vi "Assert Trigger.vi"(8 "error in (no error)":errorcluster, 9 "Trigger Number (1)":i32=1, 10 "Trigger Type (3: Trigger Generator)":i32(ring)=3 items=["Digital IO", "TSP Link", "LAN", "Trigger Generator"], 11 "VISA resource name":refnum<visa-resource-name>) -> (0 "error out":errorcluster, 3 "VISA resource name out":refnum<visa-resource-name>)   [LabVIEW 2020, in "Keithley 2600 Series.lvlib"]
doc: "Asserts a trigger and generates the corresponding event ID."
uses:
  <instrlib>/Keithley 2600 Series/Keithley 2600 Series.lvlib
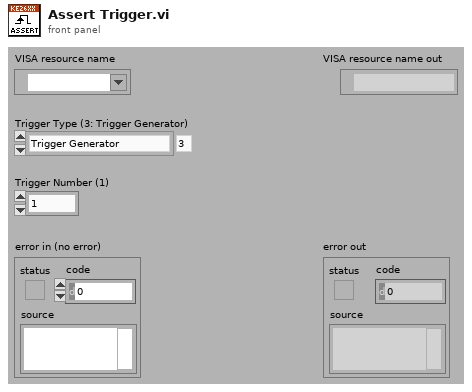
[diagram p1: front panel]
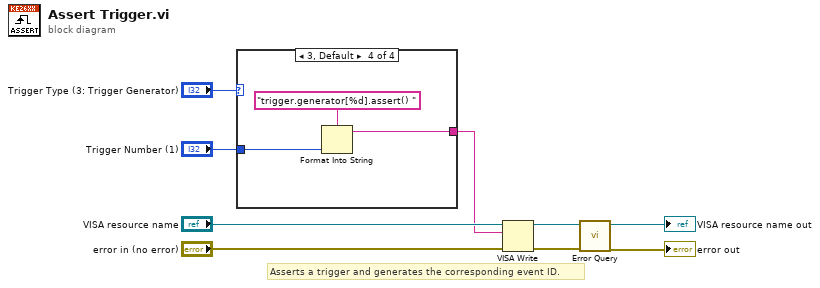
[diagram p0: block diagram]
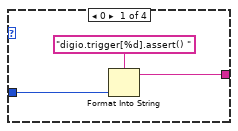
[diagram p2: hidden frame]
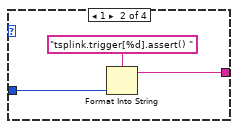
[diagram p3: hidden frame]
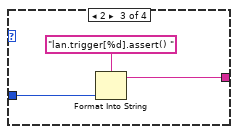
[diagram p4: hidden frame]
diagram:
  # "Asserts a trigger and generates the corresponding event ID."
  n1 = case shown="3, Default" "Trigger Type (3: Trigger Generator)" {
    tunnel: "Trigger Number (1)" -> [w11 w14 w17 w20]
    tunnel: [w10 w13 w16 w19] -> w1
    frame 0 {
      n2 = Format Into String(format string="digio.trigger[%d].assert() ", w11) -> (resulting string=w10:string)  [unwired: 2 in, 1 out]
    }
    frame 1 {
      n3 = Format Into String(format string="tsplink.trigger[%d].assert() ", w14) -> (resulting string=w13:string)  [unwired: 2 in, 1 out]
    }
    frame 2 {
      n4 = Format Into String(format string="lan.trigger[%d].assert() ", w17) -> (resulting string=w16:string)  [unwired: 2 in, 1 out]
    }
    frame 3, Default {
      n5 = Format Into String(format string="trigger.generator[%d].assert() ", w20) -> (resulting string=w19:string)  [unwired: 2 in, 1 out]
    }
  }
  n6 = VISA Write(VISA resource name="VISA resource name", write buffer=w1, error in (no error)="error in (no error)") -> (VISA resource name out=w7:refnum<visa-resource-name>, error out=w6:errorcluster)  [unwired: 1 out]
  n7 = call <instrlib>:"Error Query.vi"("error in (no error)"=w6, "VISA resource name"=w7) -> ("error out"=→"error out":errorcluster, "VISA resource name out"=→"VISA resource name out":refnum<visa-resource-name>)  [unwired: 6 in, 2 out]
